vi "transfer_and_submit_job.vi"(8 "error in (no error)":errorcluster, 9 "Password":string, 10 "Username":string, 11 "Experiment Folder":string) -> (0 "error out":errorcluster)   [LabVIEW 2019]
uses:
  ParametersGlobal.vi
panel:
  out "standard error":string
  out "standard output":string
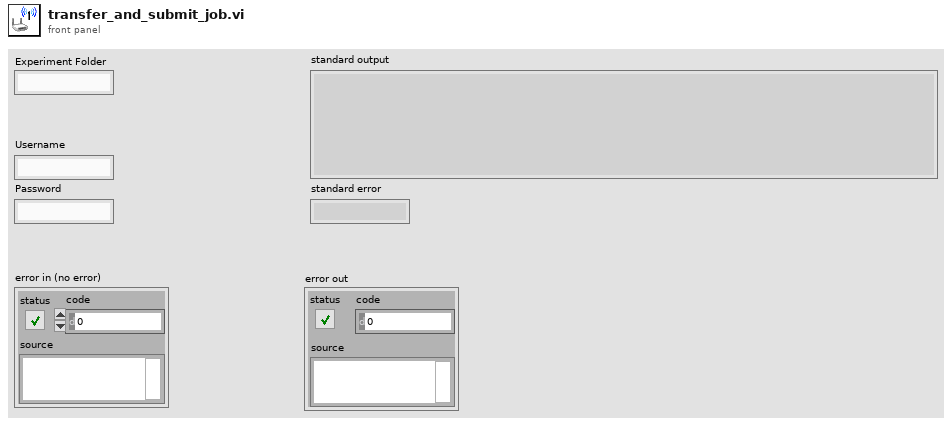
[diagram p1: front panel]
types:
  T1 = enum16{"open", "replace", "create", "open or create", "replace or create", "replace or create with confirmation"}
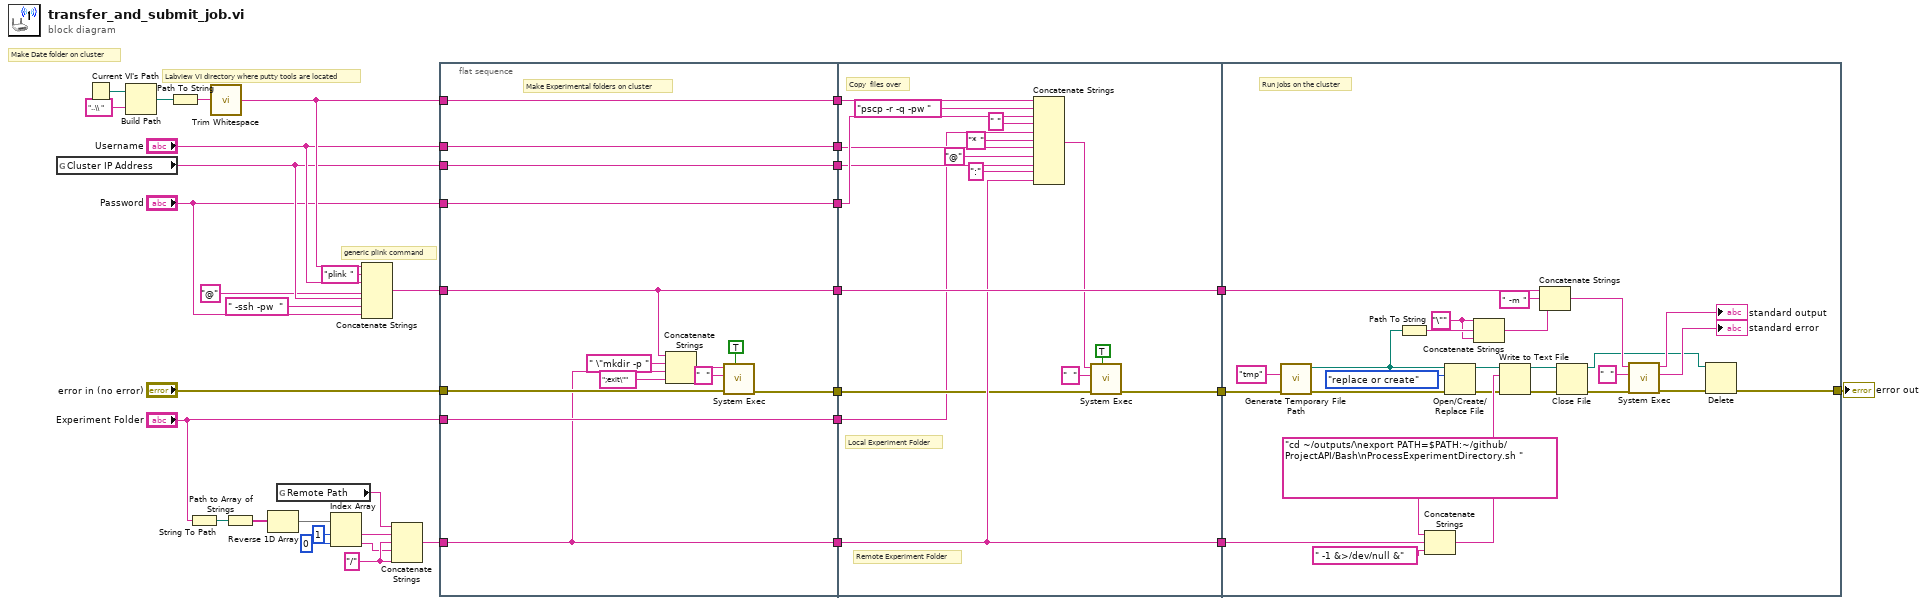
[diagram p0: block diagram]
diagram:
  w5 = "/"
  # "generic plink command"
  # "Make Date folder on cluster"
  # "Labview VI directory where putty tools are located"
  n1 = global read "ParametersGlobal.vi" "Cluster IP Address"() -> (w22:string)
  n2 = Current VI's Path() -> (path=w16:path)
  n3 = Build Path(base path=w16, name or relative path="..\\ ") -> (appended path=w18:path)
  n4 = Path To String(path=w18) -> (string=w19:string)
  n5 = String To Path(string="Experiment Folder") -> (path=w11:path)
  n6 = call <vilib>:"Trim Whitespace.vi"("string"=w19) -> ("trimmed string"=w24:string)  [unwired: 1 in]
  n7 = Path to Array of Strings(0:w11) -> (2:w8:string[])  [unwired: 1 out]
  n8 = Reverse 1D Array(array=w8) -> (reversed array=w7:string[])
  n9 = global read "ParametersGlobal.vi" "Remote Path"() -> (w12:string)
  n10 = Index Array(array=w7, index #1=1 ("index"), index #2=0 ("index")) -> (element #1=w2:string, element #2=w1:string)
  n11 = Concatenate Strings(w24, "plink ", "Username", "@", w22, " -ssh -pw  ", "Password") -> (w20:string)
  n12 = Concatenate Strings(w12, w2, w5, w1, w5) -> (w6:string)
  n13 = flat-sequence {
    tunnel: [w43] -> w34
    tunnel: [w41] -> w33
    tunnel: [w42] -> w32
    tunnel: [w49] -> w31
    tunnel: w24 -> [w49]
    tunnel: [w37] -> w30
    tunnel: [w40] -> w29
    tunnel: [w44] -> w28
    tunnel: "Username" -> [w43]
    tunnel: w22 -> [w42]
    tunnel: "Password" -> [w41]
    tunnel: w20 -> [w40]
    tunnel: "error in (no error)" -> [w39]
    tunnel: "Experiment Folder" -> [w38]
    tunnel: [w38] -> w9
    tunnel: w6 -> [w37]
    tunnel: w34 -> [w60]
    tunnel: w33 -> [w64]
    tunnel: w32 -> [w59]
    tunnel: w31 -> [w65]
    tunnel: [w57] -> w27
    tunnel: w30 -> [w57]
    tunnel: [w67] -> w26
    tunnel: w29 -> [w67]
    tunnel: w28 -> [w53]
    tunnel: [w52] -> w25
    tunnel: w9 -> [w51]
    tunnel: w27 -> [w74]
    tunnel: w26 -> [w73]
    tunnel: w25 -> [w72]
    tunnel: [w69] -> w35
    frame #0 {
      # "Make Experimental folders on cluster"
      n14 = Concatenate Strings(w40, " \"mkdir -p ", w37, ";exit\"") -> (w45:string)
      n15 = call <vilib>:"System Exec.vi"("wait until completion? (T)"=TRUE, "error in (no error)"=w39, "standard input"="  ", "command line"=w45) -> ("error out"=w44:errorcluster)  [unwired: 4 in, 3 out]
    }
    frame #1 {
      # "Remote Experiment Folder"
      # "Local Experiment Folder"
      # "Copy  files over"
      n16 = Concatenate Strings(w65, "pscp -r -q -pw ", w64, " ", w51, "* ", w60, "@", w59, ":", w57) -> (w54:string)
      n17 = call <vilib>:"System Exec.vi"("wait until completion? (T)"=TRUE, "error in (no error)"=w53, "standard input"="  ", "command line"=w54) -> ("error out"=w52:errorcluster)  [unwired: 4 in, 3 out]
    }
    frame #2 {
      w70 = "\""
      # "Run jobs on the cluster"
      n18 = call <vilib>:"Generate Temporary File Path.vi"("error in (no error)"=w72, "Temporary File Extension (tmp)"="tmp") -> ("error out"=w80:errorcluster, "Unique Temporary File Path"=w86:path)  [unwired: 8 in]
      n19 = Path To String(path=w86) -> (string=w71:string)
      n20 = Concatenate Strings("cd ~/outputs/\nexport PATH=$PATH:~/github/ProjectAPI/Bash\nProcessExperimentDirectory.sh ", w74, " -1 &>/dev/null &") -> (w87:string)
      n21 = Open/Create/Replace File(file path (use dialog)=w86, error in=w80, operation (0:open)=T1."replace or create") -> (refnum out=w81:refnum<file>, error out=w78:errorcluster)  [unwired: 3 in, 1 out]
      n22 = Concatenate Strings(w70, w71, w70) -> (w77:string)
      n23 = Write to Text File(file (use dialog)=w81, text=w87, error in=w78) -> (refnum out=w82:refnum<file>, error out=w79:errorcluster)  [unwired: 1 in, 1 out]
      n24 = Concatenate Strings(w73, " -m ", w77) -> (w88:string)
      n25 = Close File(refnum=w82, error in=w79) -> (error out=w83:errorcluster)  [unwired: 1 out]
      n26 = call <vilib>:"System Exec.vi"("error in (no error)"=w83, "standard input"="  ", "command line"=w88) -> ("error out"=w84:errorcluster, "standard error"=→"standard error":string, "standard output"=→"standard output":string)  [unwired: 5 in, 1 out]
      n27 = Delete(path (use dialog)=w86, error in=w84) -> (error out=w69:errorcluster)  [unwired: 3 in, 2 out]
    }
  }
  "error out" <- w35
